vi "Untitled 1.vi"() -> ()   [LabVIEW 2017]
uses:
  JSONtext.lvlib
panel:
  out "error out 2":errorcluster
  out "Variant out":variant
  out "error out":errorcluster
  out "value":dbl[][](array[numeric])
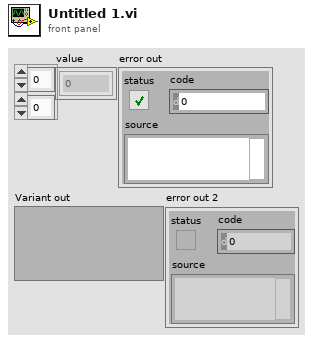
[diagram p1: front panel]
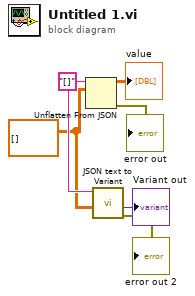
[diagram p0: block diagram]
diagram:
  w3 = dbl[][] []
  w4 = "[]" ("JSON string")
  n1 = Unflatten From JSON(JSON string=w4, type and defaults=w3) -> (value=→"value":dbl[][], error out=→"error out":errorcluster)  [unwired: 5 in]
  n2 = call "JSON text to Variant.vi"("Data Type"=w3, "JSON"=w4) -> ("error out"=→"error out 2":errorcluster, "Variant out"=→"Variant out":variant)  [unwired: 8 in]
